vi "保存判定Title文件.vi"(9 "基路径":path) -> (0 "Title":string[](array[string]), 1 "侧面":path, 2 "正面":path, 3 "路径":path, 4 "dup path":path, 5 "Title2":string[](array[string]), 7 "路径 2":path)   [LabVIEW 2017]
uses:
  <vilib>/Utility/file.llb/Read From Spreadsheet File (string).vi
  <vilib>/Utility/file.llb/Write To Spreadsheet File (string).vi
panel:
  out "侧面 8":path
  out "侧面 7":path
  out "侧面 6":path
  out "侧面 5":path
  out "Title 2":string[](array[string])
  out "添加的路径 2":path
  out "侧面 4":path
  out "侧面 3":path
  out "侧面 2":path
  out "添加的路径":path
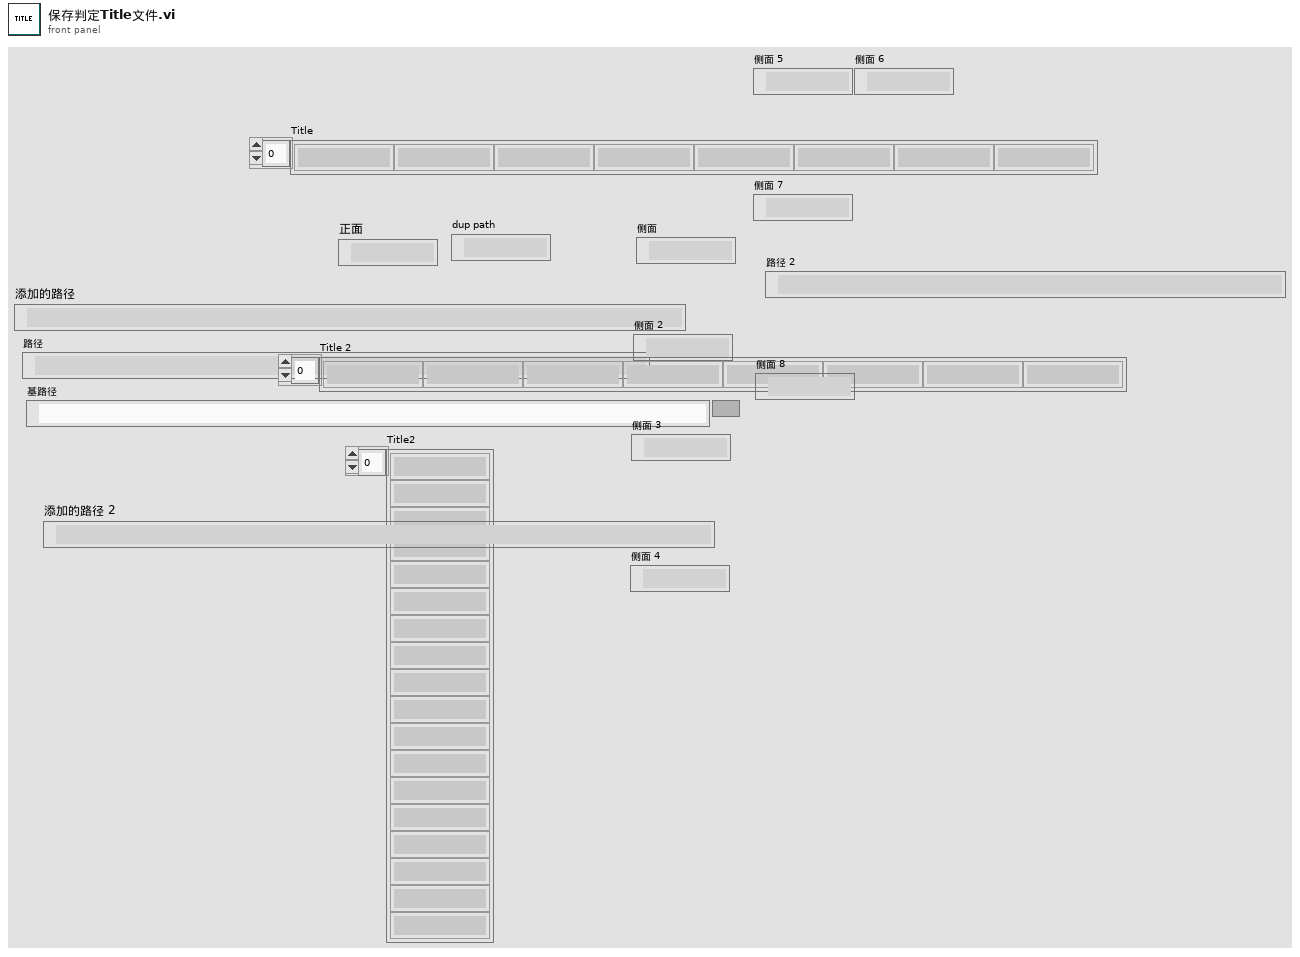
[diagram p1: front panel]
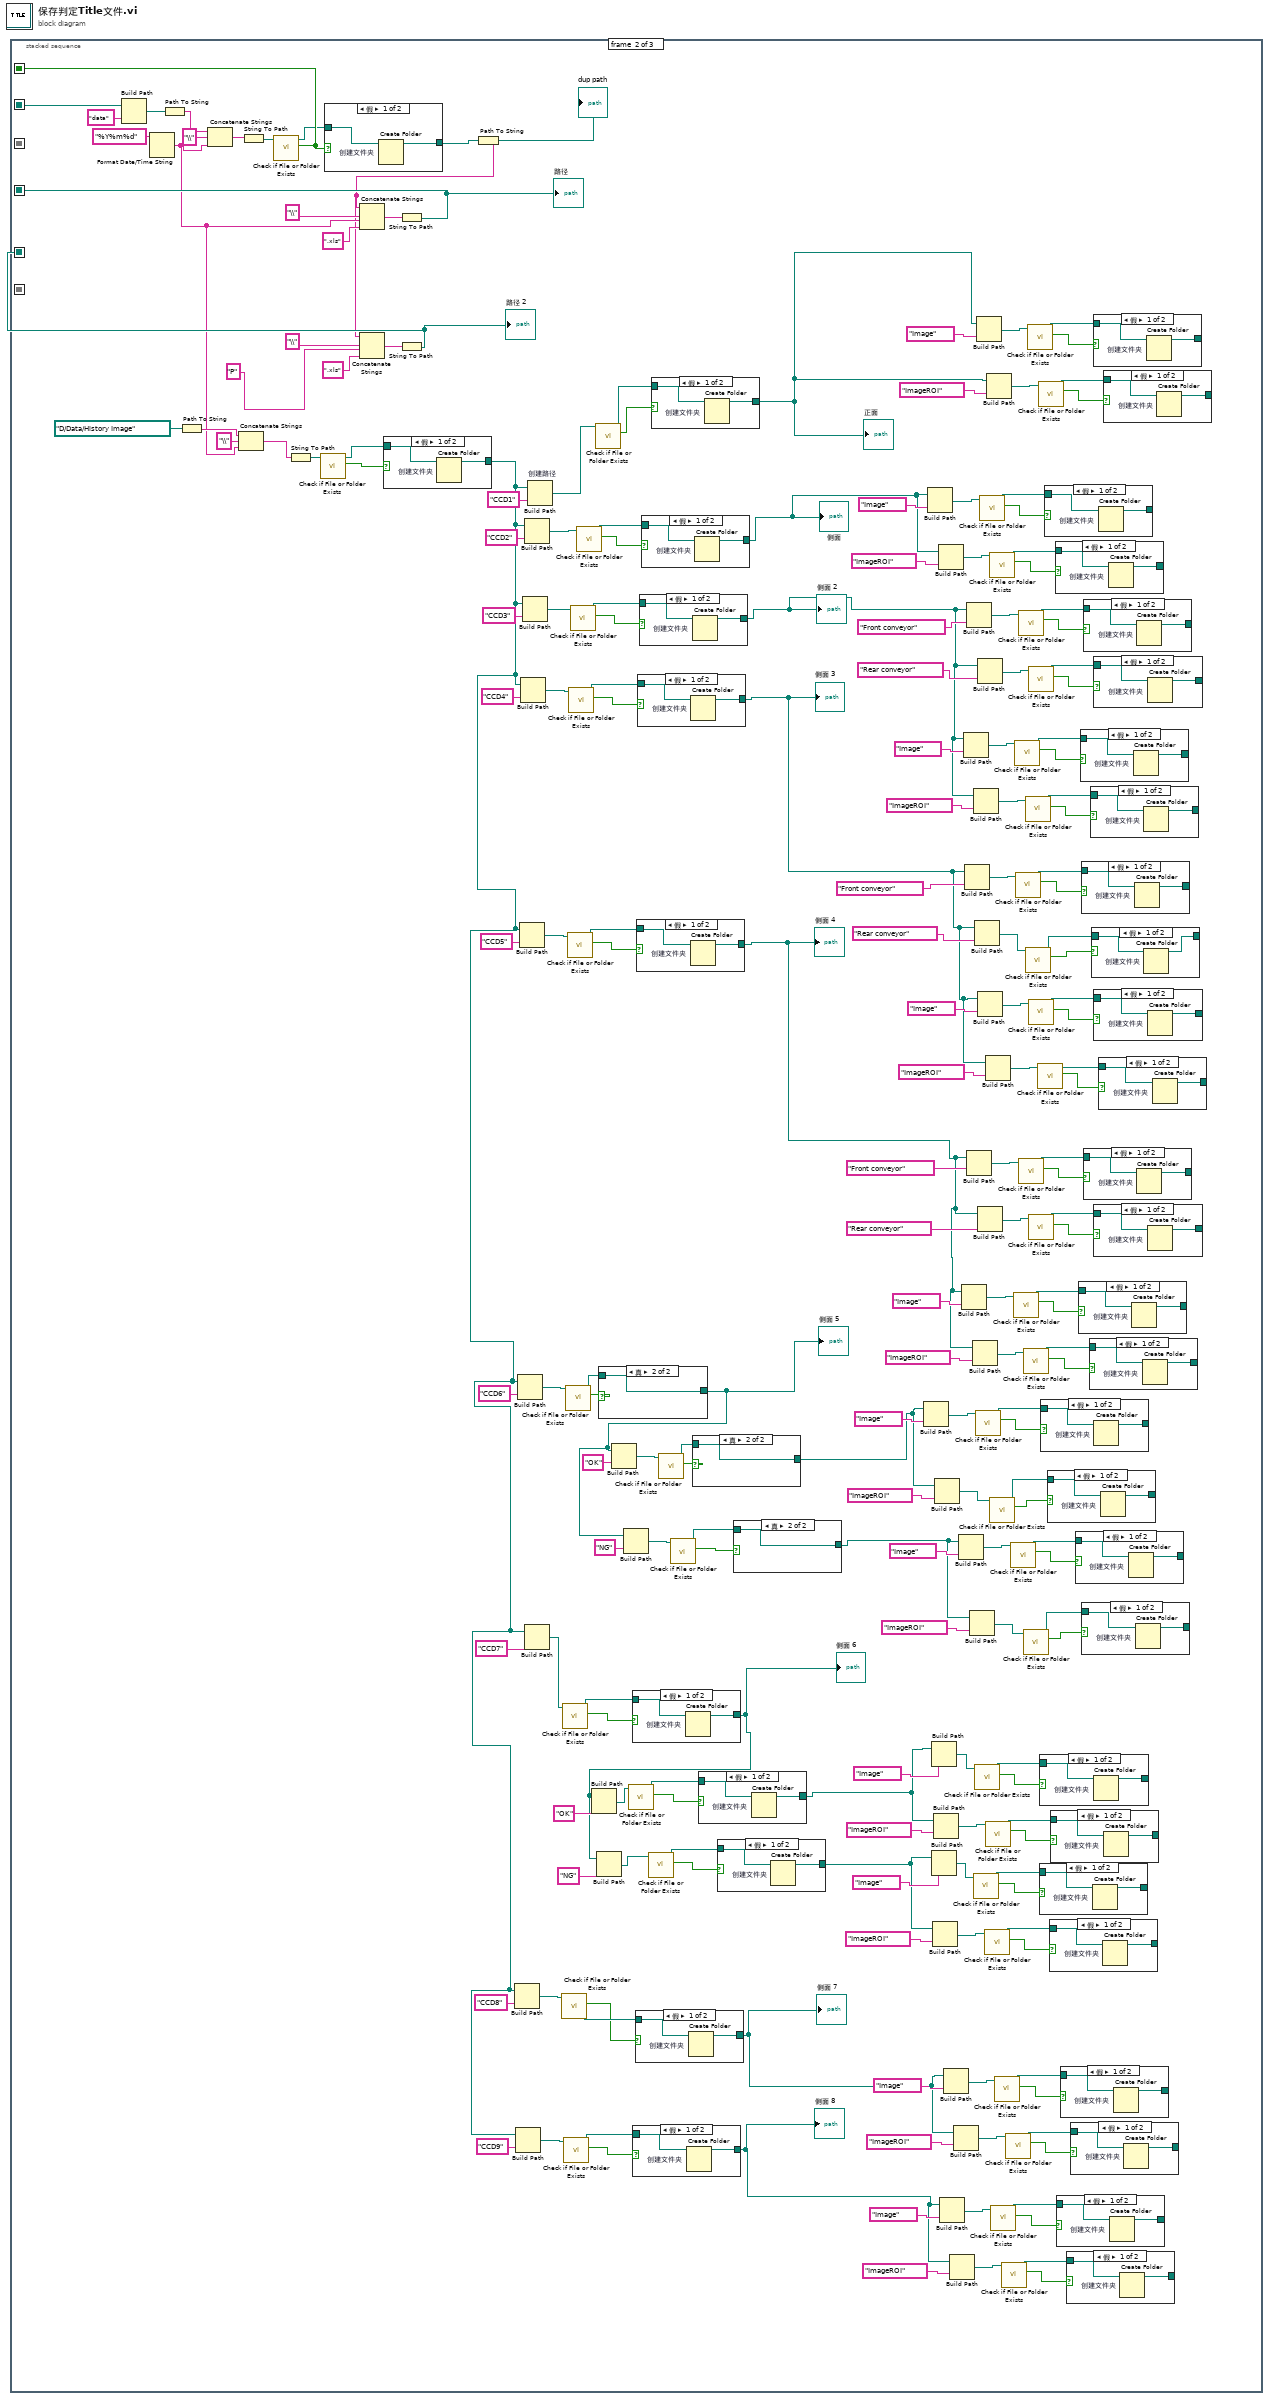
[diagram p0: block diagram]
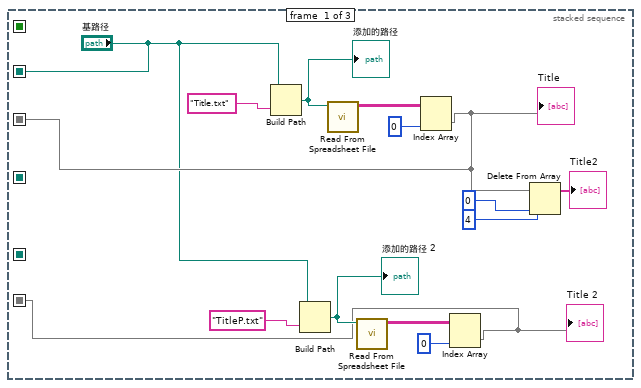
[diagram p2: hidden frame]
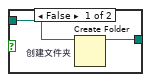
[diagram p7: hidden frame]
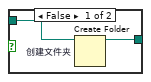
[diagram p8: hidden frame]
diagram:
  n1 = stacked-sequence {
    seq-local: ["基路径" _ _] -> [_ w211 _]
    seq-local: [_ w210 _] -> [_ _ w355]
    seq-local: [w11 _ _] -> [_ _ w353]
    seq-local: [_ w112 _] -> [_ _ w352]
    seq-local: [_ w107 _] -> [_ _ w354]
    seq-local: [w1 _ _] -> [_ _ w351]
    frame #0 {
      n2 = Build Path(base path="基路径", name or relative path="Title.txt" ("名称或相对路径")) -> (appended path=w13:path)
      "添加的路径" <- w13
      n3 = Build Path(base path="基路径", name or relative path="TitleP.txt" ("名称或相对路径")) -> (appended path=w4:path)
      "添加的路径 2" <- w4
      n4 = call-poly <vilib>:"Read From Spreadsheet File.vi"("file path (dialog if empty)"=w13) -> ("all rows"=w12:string[][])  [unwired: 6 in, 4 out]
      n5 = call-poly <vilib>:"Read From Spreadsheet File.vi"("file path (dialog if empty)"=w4) -> ("all rows"=w5:string[][])  [unwired: 6 in, 4 out]
      n6 = Index Array(array=w12, index (col)=0 ("禁用的索引 (列)")) -> (element=w11:string[])  [unwired: 1 in]
      "Title" <- w11
      n7 = Index Array(array=w5, index (col)=0 ("禁用的索引 (列)")) -> (element=w1:string[])  [unwired: 1 in]
      "Title 2" <- w1
      n8 = Delete From Array(array=w11, length=4 ("长度"), index=0 ("索引")) -> (array with subset deleted=→"Title2":string[])  [unwired: 1 out]
    }
    frame #1 {
      n9 = Build Path(base path=w211, name or relative path="data" ("名称或相对路径")) -> (appended path=w219:path)
      n10 = Format Date/Time String(time format string (%c)="%Y%m%d" ("时间格式字符串(%c)")) -> (date/time string=w106:string)  [unwired: 2 in]
      n11 = Path To String(path=w219) -> (string=w218:string)
      n12 = Path To String(path=path "D:/Data/History Image" ("添加的路径")) -> (string=w208:string)
      n13 = Concatenate Strings(w218, "\\" ("字符串"), w106) -> (w113:string)
      n14 = Concatenate Strings(w208, "\\" ("字符串"), w106) -> (w204:string)
      n15 = String To Path(string=w113) -> (path=w216:path)
      n16 = call <vilib>:"Check if File or Folder Exists.vi"("path"=w216) -> ("file or folder exists?"=w112:bool, "dup path"=w111:path)  [unwired: 8 in, 1 out]
      n17 = String To Path(string=w204) -> (path=w205:path)
      n18 = call <vilib>:"Check if File or Folder Exists.vi"("path"=w205) -> ("file or folder exists?"=w203:bool, "dup path"=w206:path)  [unwired: 8 in, 1 out]
      n19 = case shown="假" w112 {
        tunnel: w111 -> [w349 w350]
        tunnel: [w348 w350] -> w212
        frame False {
          n20 = Create Folder "创建文件夹"(path (use dialog)=w349) -> (created path=w348:path)  [unwired: 2 in, 2 out]
        }
        frame True {
        }
      }
      "dup path" <- w212
      n21 = case shown="假" w203 {
        tunnel: w206 -> [w346 w347]
        tunnel: [w345 w347] -> w62
        frame False {
          n22 = Create Folder "创建文件夹"(path (use dialog)=w346) -> (created path=w345:path)  [unwired: 2 in, 2 out]
        }
        frame True {
        }
      }
      n23 = Path To String(path=w212) -> (string=w105:string)
      n24 = Concatenate Strings(w105, "\\" ("字符串"), w106, ".xls" ("字符串")) -> (w213:string)
      n25 = Concatenate Strings(w105, "\\" ("字符串"), "P" ("字符串"), ".xls" ("字符串")) -> (w110:string)
      n26 = String To Path(string=w213) -> (path=w210:path)
      "路径" <- w210
      n27 = String To Path(string=w110) -> (path=w107:path)
      "路径 2" <- w107
      n28 = Build Path(base path=w62, name or relative path="CCD8" ("名称或相对路径")) -> (appended path=w92:path)
      n29 = Build Path(base path=w62, name or relative path="CCD9" ("名称或相对路径")) -> (appended path=w66:path)
      n30 = Build Path(base path=w62, name or relative path="CCD6" ("名称或相对路径")) -> (appended path=w100:path)
      n31 = Build Path(base path=w62, name or relative path="CCD5" ("名称或相对路径")) -> (appended path=w156:path)
      n32 = Build Path(base path=w62, name or relative path="CCD4" ("名称或相对路径")) -> (appended path=w187:path)
      n33 = Build Path(base path=w62, name or relative path="CCD3" ("名称或相对路径")) -> (appended path=w194:path)
      n34 = Build Path(base path=w62, name or relative path="CCD2" ("名称或相对路径")) -> (appended path=w195:path)
      n35 = Build Path(base path=w62, name or relative path="CCD7" ("名称或相对路径")) -> (appended path=w99:path)
      n36 = Build Path "创建路径"(base path=w62, name or relative path="CCD1" ("名称或相对路径")) -> (appended path=w198:path)
      n37 = call <vilib>:"Check if File or Folder Exists.vi"("path"=w92) -> ("file or folder exists?"=w93:bool, "dup path"=w94:path)  [unwired: 8 in, 1 out]
      n38 = call <vilib>:"Check if File or Folder Exists.vi"("path"=w99) -> ("file or folder exists?"=w98:bool, "dup path"=w97:path)  [unwired: 8 in, 1 out]
      n39 = call <vilib>:"Check if File or Folder Exists.vi"("path"=w66) -> ("file or folder exists?"=w65:bool, "dup path"=w64:path)  [unwired: 8 in, 1 out]
      n40 = call <vilib>:"Check if File or Folder Exists.vi"("path"=w100) -> ("file or folder exists?"=w101:bool, "dup path"=w102:path)  [unwired: 8 in, 1 out]
      n41 = call <vilib>:"Check if File or Folder Exists.vi"("path"=w156) -> ("file or folder exists?"=w155:bool, "dup path"=w154:path)  [unwired: 8 in, 1 out]
      n42 = call <vilib>:"Check if File or Folder Exists.vi"("path"=w187) -> ("file or folder exists?"=w188:bool, "dup path"=w189:path)  [unwired: 8 in, 1 out]
      n43 = call <vilib>:"Check if File or Folder Exists.vi"("path"=w194) -> ("file or folder exists?"=w193:bool, "dup path"=w192:path)  [unwired: 8 in, 1 out]
      n44 = call <vilib>:"Check if File or Folder Exists.vi"("path"=w195) -> ("file or folder exists?"=w196:bool, "dup path"=w197:path)  [unwired: 8 in, 1 out]
      n45 = call <vilib>:"Check if File or Folder Exists.vi"("path"=w198) -> ("file or folder exists?"=w200:bool, "dup path"=w199:path)  [unwired: 8 in, 1 out]
      n46 = case shown="真" w101 {
        tunnel: w102 -> [w280 w281]
        tunnel: [w279 w281] -> w37
        frame False {
          n47 = Create Folder "创建文件夹"(path (use dialog)=w280) -> (created path=w279:path)  [unwired: 2 in, 2 out]
        }
        frame True {
        }
      }
      "侧面 5" <- w37
      n48 = Build Path(base path=w37, name or relative path="OK" ("名称或相对路径")) -> (appended path=w44:path)
      n49 = Build Path(base path=w37, name or relative path="NG" ("名称或相对路径")) -> (appended path=w39:path)
      n50 = case shown="假" w98 {
        tunnel: w97 -> [w277 w278]
        tunnel: [w276 w278] -> w17
        frame False {
          n51 = Create Folder "创建文件夹"(path (use dialog)=w277) -> (created path=w276:path)  [unwired: 2 in, 2 out]
        }
        frame True {
        }
      }
      "侧面 6" <- w17
      n52 = Build Path(base path=w17, name or relative path="OK" ("名称或相对路径")) -> (appended path=w19:path)
      n53 = Build Path(base path=w17, name or relative path="NG" ("名称或相对路径")) -> (appended path=w18:path)
      n54 = call <vilib>:"Check if File or Folder Exists.vi"("path"=w19) -> ("file or folder exists?"=w24:bool, "dup path"=w25:path)  [unwired: 8 in, 1 out]
      n55 = case shown="假" w65 {
        tunnel: w64 -> [w253 w254]
        tunnel: [w252 w254] -> w53
        frame False {
          n56 = Create Folder "创建文件夹"(path (use dialog)=w253) -> (created path=w252:path)  [unwired: 2 in, 2 out]
        }
        frame True {
        }
      }
      "侧面 8" <- w53
      n57 = case shown="假" w93 {
        tunnel: w94 -> [w274 w275]
        tunnel: [w273 w275] -> w67
        frame False {
          n58 = Create Folder "创建文件夹"(path (use dialog)=w274) -> (created path=w273:path)  [unwired: 2 in, 2 out]
        }
        frame True {
        }
      }
      "侧面 7" <- w67
      n59 = case shown="假" w155 {
        tunnel: w154 -> [w307 w308]
        tunnel: [w306 w308] -> w114
        frame False {
          n60 = Create Folder "创建文件夹"(path (use dialog)=w307) -> (created path=w306:path)  [unwired: 2 in, 2 out]
        }
        frame True {
        }
      }
      "侧面 4" <- w114
      n61 = case shown="假" w188 {
        tunnel: w189 -> [w334 w335]
        tunnel: [w333 w335] -> w115
        frame False {
          n62 = Create Folder "创建文件夹"(path (use dialog)=w334) -> (created path=w333:path)  [unwired: 2 in, 2 out]
        }
        frame True {
        }
      }
      "侧面 3" <- w115
      n63 = case shown="假" w193 {
        tunnel: w192 -> [w337 w338]
        tunnel: [w336 w338] -> w116
        frame False {
          n64 = Create Folder "创建文件夹"(path (use dialog)=w337) -> (created path=w336:path)  [unwired: 2 in, 2 out]
        }
        frame True {
        }
      }
      "侧面 2" <- w116
      n65 = case shown="假" w196 {
        tunnel: w197 -> [w340 w341]
        tunnel: [w339 w341] -> w178
        frame False {
          n66 = Create Folder "创建文件夹"(path (use dialog)=w340) -> (created path=w339:path)  [unwired: 2 in, 2 out]
        }
        frame True {
        }
      }
      "侧面" <- w178
      n67 = call <vilib>:"Check if File or Folder Exists.vi"("path"=w18) -> ("file or folder exists?"=w23:bool, "dup path"=w22:path)  [unwired: 8 in, 1 out]
      n68 = case shown="假" w200 {
        tunnel: w199 -> [w343 w344]
        tunnel: [w342 w344] -> w157
        frame False {
          n69 = Create Folder "创建文件夹"(path (use dialog)=w343) -> (created path=w342:path)  [unwired: 2 in, 2 out]
        }
        frame True {
        }
      }
      "正面" <- w157
      n70 = call <vilib>:"Check if File or Folder Exists.vi"("path"=w44) -> ("file or folder exists?"=w43:bool, "dup path"=w42:path)  [unwired: 8 in, 1 out]
      n71 = call <vilib>:"Check if File or Folder Exists.vi"("path"=w39) -> ("file or folder exists?"=w40:bool, "dup path"=w41:path)  [unwired: 8 in, 1 out]
      n72 = case shown="真" w43 {
        tunnel: w42 -> [w238 w239]
        tunnel: [w237 w239] -> w34
        frame False {
          n73 = Create Folder "创建文件夹"(path (use dialog)=w238) -> (created path=w237:path)  [unwired: 2 in, 2 out]
        }
        frame True {
        }
      }
      n74 = case shown="假" w24 {
        tunnel: w25 -> [w226 w227]
        tunnel: [w225 w227] -> w16
        frame False {
          n75 = Create Folder "创建文件夹"(path (use dialog)=w226) -> (created path=w225:path)  [unwired: 2 in, 2 out]
        }
        frame True {
        }
      }
      n76 = case shown="假" w23 {
        tunnel: w22 -> [w223 w224]
        tunnel: [w222 w224] -> w15
        frame False {
          n77 = Create Folder "创建文件夹"(path (use dialog)=w223) -> (created path=w222:path)  [unwired: 2 in, 2 out]
        }
        frame True {
        }
      }
      n78 = case shown="真" w40 {
        tunnel: w41 -> [w235 w236]
        tunnel: [w234 w236] -> w35
        frame False {
          n79 = Create Folder "创建文件夹"(path (use dialog)=w235) -> (created path=w234:path)  [unwired: 2 in, 2 out]
        }
        frame True {
        }
      }
      n80 = Build Path(base path=w34, name or relative path="Image" ("类型")) -> (appended path=w84:path)
      n81 = Build Path(base path=w178, name or relative path="Image" ("类型")) -> (appended path=w186:path)
      n82 = Build Path(base path=w15, name or relative path="Image" ("类型")) -> (appended path=w26:path)
      n83 = Build Path(base path=w16, name or relative path="Image" ("类型")) -> (appended path=w83:path)
      n84 = Build Path(base path=w15, name or relative path="ImageROI" ("类型")) -> (appended path=w33:path)
      n85 = Build Path(base path=w16, name or relative path="ImageROI" ("类型")) -> (appended path=w76:path)
      n86 = Build Path(base path=w34, name or relative path="ImageROI" ("类型")) -> (appended path=w91:path)
      n87 = Build Path(base path=w178, name or relative path="ImageROI" ("类型")) -> (appended path=w179:path)
      n88 = Build Path(base path=w53, name or relative path="Image" ("类型")) -> (appended path=w61:path)
      n89 = Build Path(base path=w67, name or relative path="Image" ("类型")) -> (appended path=w68:path)
      n90 = Build Path(base path=w53, name or relative path="ImageROI" ("类型")) -> (appended path=w54:path)
      n91 = Build Path(base path=w67, name or relative path="ImageROI" ("类型")) -> (appended path=w75:path)
      n92 = Build Path(base path=w35, name or relative path="Image" ("类型")) -> (appended path=w52:path)
      n93 = Build Path(base path=w114, name or relative path="Image" ("类型")) -> (appended path=w124:path)
      n94 = Build Path(base path=w116, name or relative path="Image" ("类型")) -> (appended path=w140:path)
      n95 = Build Path(base path=w115, name or relative path="Front conveyor" ("类型")) -> (appended path=w171:path)
      n96 = Build Path(base path=w116, name or relative path="Front conveyor" ("类型")) -> (appended path=w172:path)
      n97 = Build Path(base path=w114, name or relative path="Front conveyor" ("类型")) -> (appended path=w147:path)
      n98 = Build Path(base path=w35, name or relative path="ImageROI" ("类型")) -> (appended path=w45:path)
      n99 = Build Path(base path=w114, name or relative path="ImageROI" ("类型")) -> (appended path=w117:path)
      n100 = Build Path(base path=w116, name or relative path="ImageROI" ("类型")) -> (appended path=w133:path)
      n101 = call <vilib>:"Check if File or Folder Exists.vi"("path"=w26) -> ("file or folder exists?"=w27:bool, "dup path"=w28:path)  [unwired: 8 in, 1 out]
      n102 = Build Path(base path=w115, name or relative path="Rear conveyor" ("类型")) -> (appended path=w166:path)
      n103 = call <vilib>:"Check if File or Folder Exists.vi"("path"=w83) -> ("file or folder exists?"=w82:bool, "dup path"=w81:path)  [unwired: 8 in, 1 out]
      n104 = call <vilib>:"Check if File or Folder Exists.vi"("path"=w84) -> ("file or folder exists?"=w85:bool, "dup path"=w86:path)  [unwired: 8 in, 1 out]
      n105 = Build Path(base path=w157, name or relative path="Image" ("类型")) -> (appended path=w158:path)
      n106 = Build Path(base path=w116, name or relative path="Rear conveyor" ("类型")) -> (appended path=w177:path)
      n107 = Build Path(base path=w115, name or relative path="Image" ("类型")) -> (appended path=w132:path)
      n108 = Build Path(base path=w114, name or relative path="Rear conveyor" ("类型")) -> (appended path=w152:path)
      n109 = call <vilib>:"Check if File or Folder Exists.vi"("path"=w186) -> ("file or folder exists?"=w185:bool, "dup path"=w184:path)  [unwired: 8 in, 1 out]
      n110 = call <vilib>:"Check if File or Folder Exists.vi"("path"=w33) -> ("file or folder exists?"=w32:bool, "dup path"=w31:path)  [unwired: 8 in, 1 out]
      n111 = call <vilib>:"Check if File or Folder Exists.vi"("path"=w76) -> ("file or folder exists?"=w77:bool, "dup path"=w78:path)  [unwired: 8 in, 1 out]
      n112 = Build Path(base path=w115, name or relative path="ImageROI" ("类型")) -> (appended path=w125:path)
      n113 = Build Path(base path=w157, name or relative path="ImageROI" ("类型")) -> (appended path=w165:path)
      n114 = call <vilib>:"Check if File or Folder Exists.vi"("path"=w91) -> ("file or folder exists?"=w90:bool, "dup path"=w89:path)  [unwired: 8 in, 1 out]
      n115 = call <vilib>:"Check if File or Folder Exists.vi"("path"=w179) -> ("file or folder exists?"=w180:bool, "dup path"=w181:path)  [unwired: 8 in, 1 out]
      n116 = call <vilib>:"Check if File or Folder Exists.vi"("path"=w61) -> ("file or folder exists?"=w60:bool, "dup path"=w59:path)  [unwired: 8 in, 1 out]
      n117 = call <vilib>:"Check if File or Folder Exists.vi"("path"=w68) -> ("file or folder exists?"=w69:bool, "dup path"=w70:path)  [unwired: 8 in, 1 out]
      n118 = call <vilib>:"Check if File or Folder Exists.vi"("path"=w54) -> ("file or folder exists?"=w55:bool, "dup path"=w56:path)  [unwired: 8 in, 1 out]
      n119 = call <vilib>:"Check if File or Folder Exists.vi"("path"=w75) -> ("file or folder exists?"=w74:bool, "dup path"=w73:path)  [unwired: 8 in, 1 out]
      n120 = call <vilib>:"Check if File or Folder Exists.vi"("path"=w52) -> ("file or folder exists?"=w51:bool, "dup path"=w50:path)  [unwired: 8 in, 1 out]
      n121 = call <vilib>:"Check if File or Folder Exists.vi"("path"=w124) -> ("file or folder exists?"=w123:bool, "dup path"=w122:path)  [unwired: 8 in, 1 out]
      n122 = call <vilib>:"Check if File or Folder Exists.vi"("path"=w140) -> ("file or folder exists?"=w139:bool, "dup path"=w138:path)  [unwired: 8 in, 1 out]
      n123 = call <vilib>:"Check if File or Folder Exists.vi"("path"=w171) -> ("file or folder exists?"=w170:bool, "dup path"=w169:path)  [unwired: 8 in, 1 out]
      n124 = call <vilib>:"Check if File or Folder Exists.vi"("path"=w172) -> ("file or folder exists?"=w173:bool, "dup path"=w174:path)  [unwired: 8 in, 1 out]
      n125 = call <vilib>:"Check if File or Folder Exists.vi"("path"=w147) -> ("file or folder exists?"=w148:bool, "dup path"=w149:path)  [unwired: 8 in, 1 out]
      n126 = call <vilib>:"Check if File or Folder Exists.vi"("path"=w117) -> ("file or folder exists?"=w118:bool, "dup path"=w119:path)  [unwired: 8 in, 1 out]
      n127 = call <vilib>:"Check if File or Folder Exists.vi"("path"=w45) -> ("file or folder exists?"=w46:bool, "dup path"=w47:path)  [unwired: 8 in, 1 out]
      n128 = call <vilib>:"Check if File or Folder Exists.vi"("path"=w133) -> ("file or folder exists?"=w134:bool, "dup path"=w135:path)  [unwired: 8 in, 1 out]
      n129 = call <vilib>:"Check if File or Folder Exists.vi"("path"=w166) -> ("file or folder exists?"=w167:bool, "dup path"=w168:path)  [unwired: 8 in, 1 out]
      n130 = call <vilib>:"Check if File or Folder Exists.vi"("path"=w158) -> ("file or folder exists?"=w159:bool, "dup path"=w160:path)  [unwired: 8 in, 1 out]
      n131 = call <vilib>:"Check if File or Folder Exists.vi"("path"=w177) -> ("file or folder exists?"=w176:bool, "dup path"=w175:path)  [unwired: 8 in, 1 out]
      n132 = call <vilib>:"Check if File or Folder Exists.vi"("path"=w132) -> ("file or folder exists?"=w131:bool, "dup path"=w130:path)  [unwired: 8 in, 1 out]
      n133 = call <vilib>:"Check if File or Folder Exists.vi"("path"=w152) -> ("file or folder exists?"=w151:bool, "dup path"=w150:path)  [unwired: 8 in, 1 out]
      n134 = call <vilib>:"Check if File or Folder Exists.vi"("path"=w125) -> ("file or folder exists?"=w126:bool, "dup path"=w127:path)  [unwired: 8 in, 1 out]
      n135 = call <vilib>:"Check if File or Folder Exists.vi"("path"=w165) -> ("file or folder exists?"=w164:bool, "dup path"=w163:path)  [unwired: 8 in, 1 out]
      n136 = case shown="假" w27 {
        tunnel: w28 -> [w232 w233]
        tunnel: [w231 w233] -> _
        frame False {
          n137 = Create Folder "创建文件夹"(path (use dialog)=w232) -> (created path=w231:path)  [unwired: 2 in, 2 out]
        }
        frame True {
        }
      }
      n138 = case shown="假" w82 {
        tunnel: w81 -> [w265 w266]
        tunnel: [w264 w266] -> _
        frame False {
          n139 = Create Folder "创建文件夹"(path (use dialog)=w265) -> (created path=w264:path)  [unwired: 2 in, 2 out]
        }
        frame True {
        }
      }
      n140 = case shown="假" w85 {
        tunnel: w86 -> [w271 w272]
        tunnel: [w270 w272] -> _
        frame False {
          n141 = Create Folder "创建文件夹"(path (use dialog)=w271) -> (created path=w270:path)  [unwired: 2 in, 2 out]
        }
        frame True {
        }
      }
      n142 = case shown="假" w185 {
        tunnel: w184 -> [w331 w332]
        tunnel: [w330 w332] -> _
        frame False {
          n143 = Create Folder "创建文件夹"(path (use dialog)=w331) -> (created path=w330:path)  [unwired: 2 in, 2 out]
        }
        frame True {
        }
      }
      n144 = case shown="假" w90 {
        tunnel: w89 -> [w268 w269]
        tunnel: [w267 w269] -> _
        frame False {
          n145 = Create Folder "创建文件夹"(path (use dialog)=w268) -> (created path=w267:path)  [unwired: 2 in, 2 out]
        }
        frame True {
        }
      }
      n146 = case shown="假" w32 {
        tunnel: w31 -> [w229 w230]
        tunnel: [w228 w230] -> _
        frame False {
          n147 = Create Folder "创建文件夹"(path (use dialog)=w229) -> (created path=w228:path)  [unwired: 2 in, 2 out]
        }
        frame True {
        }
      }
      n148 = case shown="假" w77 {
        tunnel: w78 -> [w262 w263]
        tunnel: [w261 w263] -> _
        frame False {
          n149 = Create Folder "创建文件夹"(path (use dialog)=w262) -> (created path=w261:path)  [unwired: 2 in, 2 out]
        }
        frame True {
        }
      }
      n150 = case shown="假" w180 {
        tunnel: w181 -> [w328 w329]
        tunnel: [w327 w329] -> _
        frame False {
          n151 = Create Folder "创建文件夹"(path (use dialog)=w328) -> (created path=w327:path)  [unwired: 2 in, 2 out]
        }
        frame True {
        }
      }
      n152 = case shown="假" w60 {
        tunnel: w59 -> [w250 w251]
        tunnel: [w249 w251] -> _
        frame False {
          n153 = Create Folder "创建文件夹"(path (use dialog)=w250) -> (created path=w249:path)  [unwired: 2 in, 2 out]
        }
        frame True {
        }
      }
      n154 = case shown="假" w69 {
        tunnel: w70 -> [w259 w260]
        tunnel: [w258 w260] -> _
        frame False {
          n155 = Create Folder "创建文件夹"(path (use dialog)=w259) -> (created path=w258:path)  [unwired: 2 in, 2 out]
        }
        frame True {
        }
      }
      n156 = case shown="假" w55 {
        tunnel: w56 -> [w247 w248]
        tunnel: [w246 w248] -> _
        frame False {
          n157 = Create Folder "创建文件夹"(path (use dialog)=w247) -> (created path=w246:path)  [unwired: 2 in, 2 out]
        }
        frame True {
        }
      }
      n158 = case shown="假" w74 {
        tunnel: w73 -> [w256 w257]
        tunnel: [w255 w257] -> _
        frame False {
          n159 = Create Folder "创建文件夹"(path (use dialog)=w256) -> (created path=w255:path)  [unwired: 2 in, 2 out]
        }
        frame True {
        }
      }
      n160 = case shown="假" w51 {
        tunnel: w50 -> [w244 w245]
        tunnel: [w243 w245] -> _
        frame False {
          n161 = Create Folder "创建文件夹"(path (use dialog)=w244) -> (created path=w243:path)  [unwired: 2 in, 2 out]
        }
        frame True {
        }
      }
      n162 = case shown="假" w123 {
        tunnel: w122 -> [w286 w287]
        tunnel: [w285 w287] -> _
        frame False {
          n163 = Create Folder "创建文件夹"(path (use dialog)=w286) -> (created path=w285:path)  [unwired: 2 in, 2 out]
        }
        frame True {
        }
      }
      n164 = case shown="假" w139 {
        tunnel: w138 -> [w298 w299]
        tunnel: [w297 w299] -> _
        frame False {
          n165 = Create Folder "创建文件夹"(path (use dialog)=w298) -> (created path=w297:path)  [unwired: 2 in, 2 out]
        }
        frame True {
        }
      }
      n166 = case shown="假" w170 {
        tunnel: w169 -> [w319 w320]
        tunnel: [w318 w320] -> _
        frame False {
          n167 = Create Folder "创建文件夹"(path (use dialog)=w319) -> (created path=w318:path)  [unwired: 2 in, 2 out]
        }
        frame True {
        }
      }
      n168 = case shown="假" w46 {
        tunnel: w47 -> [w241 w242]
        tunnel: [w240 w242] -> _
        frame False {
          n169 = Create Folder "创建文件夹"(path (use dialog)=w241) -> (created path=w240:path)  [unwired: 2 in, 2 out]
        }
        frame True {
        }
      }
      n170 = case shown="假" w173 {
        tunnel: w174 -> [w325 w326]
        tunnel: [w324 w326] -> _
        frame False {
          n171 = Create Folder "创建文件夹"(path (use dialog)=w325) -> (created path=w324:path)  [unwired: 2 in, 2 out]
        }
        frame True {
        }
      }
      n172 = case shown="假" w148 {
        tunnel: w149 -> [w304 w305]
        tunnel: [w303 w305] -> _
        frame False {
          n173 = Create Folder "创建文件夹"(path (use dialog)=w304) -> (created path=w303:path)  [unwired: 2 in, 2 out]
        }
        frame True {
        }
      }
      n174 = case shown="假" w118 {
        tunnel: w119 -> [w283 w284]
        tunnel: [w282 w284] -> _
        frame False {
          n175 = Create Folder "创建文件夹"(path (use dialog)=w283) -> (created path=w282:path)  [unwired: 2 in, 2 out]
        }
        frame True {
        }
      }
      n176 = case shown="假" w134 {
        tunnel: w135 -> [w295 w296]
        tunnel: [w294 w296] -> _
        frame False {
          n177 = Create Folder "创建文件夹"(path (use dialog)=w295) -> (created path=w294:path)  [unwired: 2 in, 2 out]
        }
        frame True {
        }
      }
      n178 = case shown="假" w167 {
        tunnel: w168 -> [w316 w317]
        tunnel: [w315 w317] -> _
        frame False {
          n179 = Create Folder "创建文件夹"(path (use dialog)=w316) -> (created path=w315:path)  [unwired: 2 in, 2 out]
        }
        frame True {
        }
      }
      n180 = case shown="假" w159 {
        tunnel: w160 -> [w313 w314]
        tunnel: [w312 w314] -> _
        frame False {
          n181 = Create Folder "创建文件夹"(path (use dialog)=w313) -> (created path=w312:path)  [unwired: 2 in, 2 out]
        }
        frame True {
        }
      }
      n182 = case shown="假" w176 {
        tunnel: w175 -> [w322 w323]
        tunnel: [w321 w323] -> _
        frame False {
          n183 = Create Folder "创建文件夹"(path (use dialog)=w322) -> (created path=w321:path)  [unwired: 2 in, 2 out]
        }
        frame True {
        }
      }
      n184 = case shown="假" w131 {
        tunnel: w130 -> [w292 w293]
        tunnel: [w291 w293] -> _
        frame False {
          n185 = Create Folder "创建文件夹"(path (use dialog)=w292) -> (created path=w291:path)  [unwired: 2 in, 2 out]
        }
        frame True {
        }
      }
      n186 = case shown="假" w151 {
        tunnel: w150 -> [w301 w302]
        tunnel: [w300 w302] -> _
        frame False {
          n187 = Create Folder "创建文件夹"(path (use dialog)=w301) -> (created path=w300:path)  [unwired: 2 in, 2 out]
        }
        frame True {
        }
      }
      n188 = case shown="假" w126 {
        tunnel: w127 -> [w289 w290]
        tunnel: [w288 w290] -> _
        frame False {
          n189 = Create Folder "创建文件夹"(path (use dialog)=w289) -> (created path=w288:path)  [unwired: 2 in, 2 out]
        }
        frame True {
        }
      }
      n190 = case shown="假" w164 {
        tunnel: w163 -> [w310 w311]
        tunnel: [w309 w311] -> _
        frame False {
          n191 = Create Folder "创建文件夹"(path (use dialog)=w310) -> (created path=w309:path)  [unwired: 2 in, 2 out]
        }
        frame True {
        }
      }
    }
    frame #2 {
      n192 = case shown="假" w352 {
        tunnel: w355 -> [w361 _]
        tunnel: w353 -> [w360 _]
        frame False {
          n193 = call-poly <vilib>:"Write To Spreadsheet File.vi"("append to file? (new file:F)"=TRUE, "1D data"=w360, "file path (dialog if empty)"=w361) -> ()  [unwired: 5 in, 1 out]
        }
        frame True {
        }
      }
      n194 = case shown="假" w352 {
        tunnel: w354 -> [w358 _]
        tunnel: w351 -> [w357 _]
        frame False {
          n195 = call-poly <vilib>:"Write To Spreadsheet File.vi"("append to file? (new file:F)"=TRUE, "1D data"=w357, "file path (dialog if empty)"=w358) -> ()  [unwired: 5 in, 1 out]
        }
        frame True {
        }
      }
    }
  }
